vi "DriveControlLoop.vi"() -> ()   [LabVIEW 2018]
uses:
  <vilib>/Rock Robotics/WPI/ThirdParty/Phoenix-LabVIEW/Motor Controller/Controls/CTRE_Phoenix_MotorControl_ControlMode.ctl
  Infrastructure/RobotMap.vi
  <vilib>/Rock Robotics/Network Tables/NT Write Number.vi
  Robot Global Data.vi
  <vilib>/Rock Robotics/WPI/ThirdParty/Phoenix-LabVIEW/Motor Controller/Get/CTRE_Phoenix_MotorController_GetSelectedSensorData.vi
  <vilib>/Rock Robotics/WPI/ThirdParty/Phoenix-LabVIEW/Motor Controller/Get/CTRE_Phoenix_MotorController_GetOutputCurrent_Enhanced.vi
  <vilib>/Rock Robotics/Network Tables/NT Write Boolean.vi
panel:
  out "MM on last step":bool
  out "Index of Current Auton Step":dbl
  out "Hab2toHab1Step":enum16{"Go Forward", "Go Backward", "Set Home"}(ring)
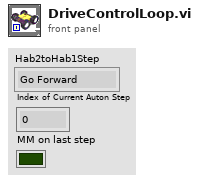
[diagram p1: front panel]
types:
  T1 = typedef "WPI_MotorControlDeviceRef.ctl" = cluster{"DeviceStatus":errorcluster, "Type":T2, "PWM":cluster{"PWM Channel":T3, "DeadBand":T4}, "CAN":cluster{"Device Number":u8, "SetOutput VI Ref":variant, "GetOutput VI Ref":variant, "Enable VI Ref":variant, "Disable VI Ref":variant, "Data":variant}, "Invert":bool, "DIO PWM":cluster{"PWM \"Enable\" Channel":T3, "DIOChannel":T5, "PWM Rate":dbl}}
  T2 = typedef "WPI_MotorControlType.ctl" = enum16{"PWM", "CAN", "DIO PWM"}
  T3 = typedef "FPGA_DIOPWMChannel.ctl" = enum8{"PWM 0", "PWM 1", "PWM 2", "PWM 3", "PWM 4", "PWM 5", "PWM 6", "PWM 7", "PWM 8", "PWM 9", "PWM MXP 0", "PWM MXP 1", "PWM MXP 2", "PWM MXP 3", "PWM MXP 4", "PWM MXP 5", "PWM MXP 6", "PWM MXP 7", "PWM MXP 8", "PWM MXP 9", "Invalid"}
  T4 = typedef "WPI_PWMDeadband.ctl" = cluster{"Name":string, "maxPositivePwm":i32, "minPositivePwm":i32, "centerPwm":i32, "maxNegativePwm":i32, "minNegativePwm":i32, "angularRange":u16}
  T5 = typedef "FPGA_DIOChannel.ctl" = enum8{"DIO 0", "DIO 1", "DIO 2", "DIO 3", "DIO 4", "DIO 5", "DIO 6", "DIO 7", "DIO 8", "DIO 9", "DIO MXP 0", "DIO MXP 1", "DIO MXP 2", "DIO MXP 3", "DIO MXP 4", "DIO MXP 5", "DIO MXP 6", "DIO MXP 7", "DIO MXP 8", "DIO MXP 9", "DIO MXP 10", "DIO MXP 11", "DIO MXP 12", "DIO MXP 13", "DIO MXP 14", "DIO MXP 15", "SPI Port CS1", "SPI Port CS2", "SPI Port CS3", "SPI Port MISO", "SPI Port MOSI", "Invalid"}
  T6 = typedef "WPI_GyroDevRef.ctl" = cluster{"DevStatus":errorcluster, "Analog Channel":T7, "Gain (VoltsPerDegree/Second)":dbl, "Gyro Type":enum16{"Analog", "XRS450"}, "Handle":i32, "SPI Bus":T8, "Device Found":bool, "Sample Rate":dbl, "Calibrate On Open":bool, "Offset":dbl}
  T7 = typedef "FPGA_AIChannel.ctl" = enum8{"AI 0", "AI 1", "AI 2", "AI 3", "AI MXP 0", "AI MXP 1", "AI MXP 2", "AI MXP 3", "Invalid"}
  T8 = typedef "spi_bus.ctl" = enum16{"SPI On-Board, CS0", "SPI On-Board, CS1", "SPI On-Board, CS2", "SPI On-Board, CS3", "SPI MXP", "Invalid"}
  T9 = cluster{"Position (Raw Sensor Units)":i32, "Velocity (Raw Sensor Units per 100 ms)":i32}
  T10 = typedef "Drive mode.ctl" = enum16{"HAB2toHAB1", "Driver Operated", "Drive Autonomously", "Disabled"}
  T11 = typedef "CTRE_Phoenix_MotorControl_ControlMode.ctl" = u16
  T12 = cluster{"Left Motor Value":dbl, "Right Motor Value":dbl}
  T13 = typedef "Drive Motion Magic Setpoints.ctl" = cluster{"Increase in Left":dbl, "Increase in Right":dbl}[]
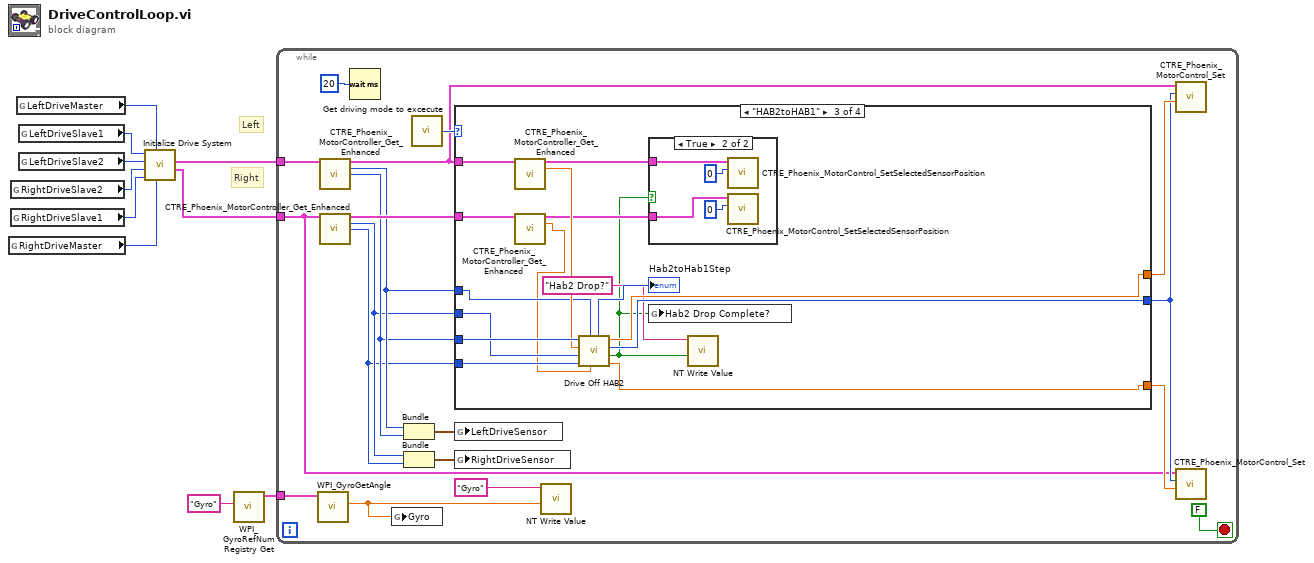
[diagram p0: block diagram]
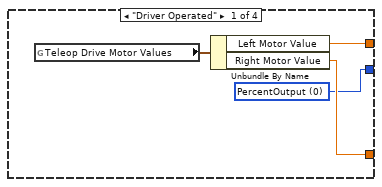
[diagram p2: hidden frame]
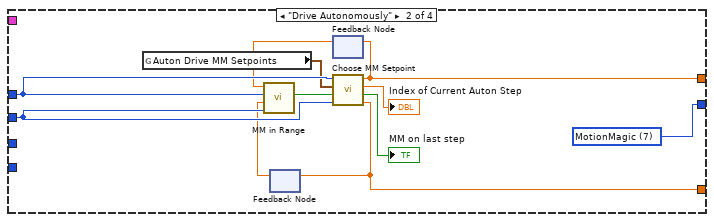
[diagram p3: hidden frame]
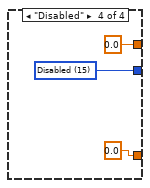
[diagram p5: hidden frame]
diagram:
  # "Right"
  # "Left"
  n1 = global read "RobotMap.vi" "RightDriveMaster"() -> (w8:u8)
  n2 = global read "RobotMap.vi" "RightDriveSlave2"() -> (w10:u8)
  n3 = global read "RobotMap.vi" "RightDriveSlave1"() -> (w9:u8)
  n4 = global read "RobotMap.vi" "LeftDriveMaster"() -> (w5:u8)
  n5 = global read "RobotMap.vi" "LeftDriveSlave1"() -> (w6:u8)
  n6 = global read "RobotMap.vi" "LeftDriveSlave2"() -> (w7:u8)
  n7 = call "Initialize Drive System.vi"("RightDriveMaster"=w8, "LeftDriveMaster"=w5, "RightDriveSlave1"=w9, "RightDriveSlave2"=w10, "LeftDriveSlave 2"=w7, "LeftDriveSlave1"=w6) -> ("RightDriveMaster"=w3:T1, "LeftDriveMaster"=w4:T1)  [unwired: 4 in]
  n8 = call <vilib>:"WPI_GyroRefNum Registry Get.vi"("refnum name"="Gyro") -> ("GyroDevRef"=w1:T6)  [unwired: 9 in, 1 out]
  n9 = while {
    tunnel: w4 -> [w16]
    tunnel: w3 -> [w15]
    tunnel: w1 -> [w23]
    stop <- FALSE stop-if-true
    n10 = call <vilib>:"WPI_GyroGetAngle.vi"("GyroDevRef"=w23) -> ("Angle"=w12:dbl)  [unwired: 6 in, 4 out]
    n11 = call-poly <vilib>:"CTRE_Phoenix_MotorController_Get_Enhanced.vi"("PhoenixMotorControlDevRef"=w16) -> ("PhoenixMotorControlDevRef"=w21:T1, "Position (Raw Sensor Units)"=w19:i32, "Velocity (Raw Sensor Units per 100 ms)"=w18:i32)  [unwired: 11 in, 1 out]
    n12 = call-poly <vilib>:"CTRE_Phoenix_MotorController_Get_Enhanced.vi"("PhoenixMotorControlDevRef"=w15) -> ("PhoenixMotorControlDevRef"=w22:T1, "Position (Raw Sensor Units)"=w14:i32, "Velocity (Raw Sensor Units per 100 ms)"=w13:i32)  [unwired: 11 in, 1 out]
    n13 = Wait (ms)(milliseconds to wait=u32 20) -> ()  [unwired: 1 out]
    n14 = global write "Robot Global Data.vi" "Gyro"(w12) -> ()
    n15 = Bundle("Position (Raw Sensor Units)"=w19, "Velocity (Raw Sensor Units per 100 ms)"=w18) -> (w20:T9)  [unwired: 1 in]
    n16 = Bundle("Position (Raw Sensor Units)"=w14, "Velocity (Raw Sensor Units per 100 ms)"=w13) -> (w17:T9)  [unwired: 1 in]
    n17 = call "Get driving mode to excecute.vi"() -> ("Drive Mode"=w24:T10)  [unwired: 1 in]
    n18 = case shown="\"HAB2toHAB1\"" w24 {
      tunnel: w19 -> [_ w43 w56 _]
      tunnel: [w32 w37 w51 0.0 ("Left Motor Value")] -> w27
      tunnel: [w30 w44 w50 w67] -> w26
      tunnel: w14 -> [_ w42 w55 _]
      tunnel: [w31 w39 w49 0.0 ("Right Motor Value")] -> w25
      tunnel: w18 -> [_ _ w58 _]
      tunnel: w13 -> [_ _ w54 _]
      tunnel: w21 -> [_ _ w60 _]
      tunnel: w22 -> [_ _ w59 _]
      frame "Driver Operated" {
        w30 = T11 0 items=["PercentOutput"=0, "Position"=1, "Velocity"=2, "Current"=3, "Follower"=5, "MotionProfile"=6, "MotionMagic"=7, "MotionProfileArc"=10, "Disabled"=15] ("Control Mode")
        n19 = global read "Robot Global Data.vi" "Teleop Drive Motor Values"() -> (w33:T12)
        n20 = Unbundle By Name(w33) -> ("Left Motor Value"=w32:dbl, "Right Motor Value"=w31:dbl)
      }
      frame "Drive Autonomously" {
        w44 = T11 7 items=["PercentOutput"=0, "Position"=1, "Velocity"=2, "Current"=3, "Follower"=5, "MotionProfile"=6, "MotionMagic"=7, "MotionProfileArc"=10, "Disabled"=15] ("Control Mode")
        n21 = global read "Robot Global Data.vi" "Auton Drive MM Setpoints"() -> (w40:T13)
        n22 = feedback #1() -> (w38:dbl)  [unwired: 1 in]
        n23 = feedback #2() -> (w36:dbl)  [unwired: 1 in]
        n24 = call "MM in Range.vi"("Right Position"=w42, "Right Setpoint"=w38, "Left position"=w43, "Left Setpoint"=w36) -> ("\"Done with step\" enough"=w41:bool)  [unwired: 7 in]
        n25 = call "Choose MM Setpoint.vi"("Right Encoder Pos"=w42, "\"Done with step\" enough"=w41, "Steps"=w40, "Left Encoder Pos"=w43) -> ("Right Motor Setpoint"=w39:dbl, "MM on last step"=→"MM on last step":bool, "Index of Current Step"=→"Index of Current Auton Step":dbl, "Left Motor Setpoint"=w37:dbl)  [unwired: 4 in]
        n26 = feedback-in #1(w39) -> ()
        n27 = feedback-in #2(w37) -> ()
      }
      frame "HAB2toHAB1" {
        n28 = call-poly <vilib>:"CTRE_Phoenix_MotorController_Get_Enhanced.vi"("PhoenixMotorControlDevRef"=w60) -> ("PhoenixMotorControlDevRef"=w48:T1, "Output Current"=w57:dbl)  [unwired: 12 in, 1 out]
        n29 = call-poly <vilib>:"CTRE_Phoenix_MotorController_Get_Enhanced.vi"("PhoenixMotorControlDevRef"=w59) -> ("PhoenixMotorControlDevRef"=w47:T1, "Output Current"=w53:dbl)  [unwired: 12 in, 1 out]
        n30 = call "Drive Off HAB2.vi"("Right Current Drawn"=w53, "Left Position"=w56, "Right Velocity"=w54, "Right Position"=w55, "Left Current Drawn"=w57, "Left Velocity"=w58) -> ("Right Output"=w49:dbl, "DONE/Zero Encoders"=w45:bool, "Control Mode"=w50:T11, "Left Output"=w51:dbl, "Step"=→"Hab2toHab1Step":enum16{"Go Forward", "Go Backward", "Set Home"})  [unwired: 1 in]
        n31 = case shown="True" w45 {
          tunnel: w48 -> [_ w62]
          tunnel: w47 -> [_ w61]
          frame False {
          }
          frame True {
            n32 = call <vilib>:"CTRE_Phoenix_MotorControl_SetSelectedSensorPosition.vi"("New Sensor Position"=0, "PhoenixMotorControlDevRef"=w62) -> ()  [unwired: 8 in, 2 out]
            n33 = call <vilib>:"CTRE_Phoenix_MotorControl_SetSelectedSensorPosition.vi"("New Sensor Position"=0, "PhoenixMotorControlDevRef"=w61) -> ()  [unwired: 8 in, 2 out]
          }
        }
        n34 = global write "Robot Global Data.vi" "Hab2 Drop Complete?"(w45) -> ()
        n35 = call-poly <vilib>:"NT Write Value.vi"("Boolean"=w45, "Name"="Hab2 Drop?") -> ()  [unwired: 9 in, 1 out]
      }
      frame "Disabled" {
        w67 = T11 15 items=["PercentOutput"=0, "Position"=1, "Velocity"=2, "Current"=3, "Follower"=5, "MotionProfile"=6, "MotionMagic"=7, "MotionProfileArc"=10, "Disabled"=15] ("Control Mode")
      }
    }
    n36 = global write "Robot Global Data.vi" "LeftDriveSensor"(w20) -> ()
    n37 = global write "Robot Global Data.vi" "RightDriveSensor"(w17) -> ()
    n38 = call-poly <vilib>:"NT Write Value.vi"("Numeric"=w12, "Name"="Gyro") -> ()  [unwired: 9 in, 1 out]
    n39 = call <vilib>:"CTRE_Phoenix_MotorControl_Set.vi"("Output"=w27, "Control Mode"=w26, "PhoenixMotorControlDevRef"=w21) -> ()  [unwired: 7 in, 2 out]
    n40 = call <vilib>:"CTRE_Phoenix_MotorControl_Set.vi"("Output"=w25, "Control Mode"=w26, "PhoenixMotorControlDevRef"=w15) -> ()  [unwired: 7 in, 2 out]
  }
